vi "Differenzzeit ermitteln.vi"(9 "Zeitstempel 2":timestamp, 11 "Zeitstempel 1":timestamp) -> (1 "Differenzzeit in ms":sgl, 2 "Differenzzeit in sec":sgl)   [LabVIEW 2020, in "LogKonfig.lvlib"]
uses:
  LogKonfig.lvlib
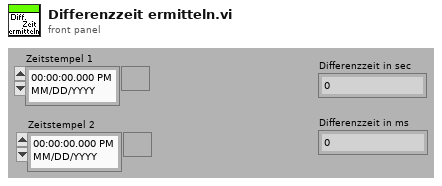
[diagram p1: front panel]
types:
  T1 = typedef "LVDateTimeRec.ctl" = cluster{"Sekundenbruchteil":dbl, "Sekunde":i32, "Minute":i32, "Stunde":i32, "Tag des Monats":i32, "Monat":i32, "Jahr":i32, "Wochentag":i32, "Tag des Jahres":i32, "DST":i32}
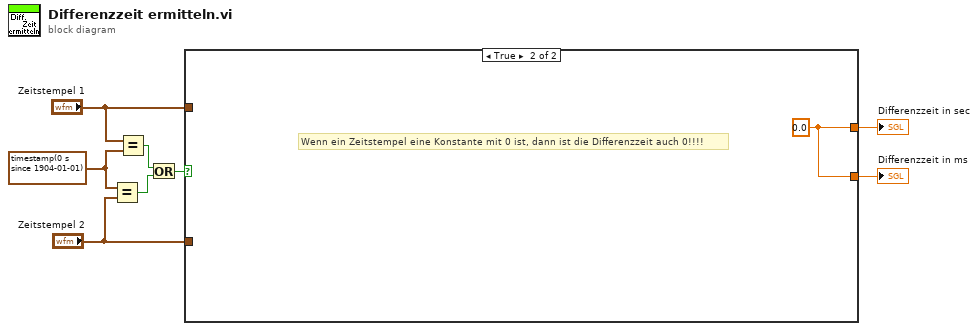
[diagram p0: block diagram]
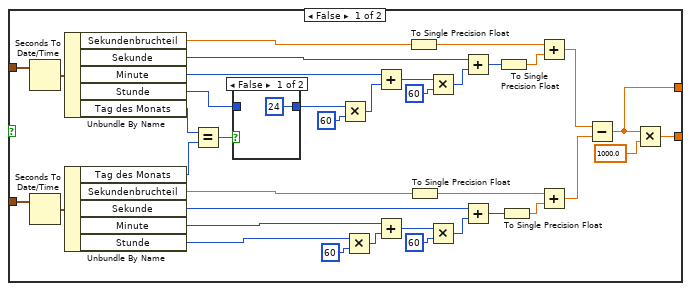
[diagram p2: hidden frame]
diagram:
  w5 = timestamp(0 s since 1904-01-01) ("Zeitstempel 2")
  n1 = Equal?(x=w5, y="Zeitstempel 2") -> (x = y?=w2:bool)
  n2 = Equal?(x="Zeitstempel 1", y=w5) -> (x = y?=w3:bool)
  n3 = Or(x=w3, y=w2) -> (x .or. y?=w1:bool)
  n4 = case shown="True" w1 {
    tunnel: [w23 w48] -> w8
    tunnel: [w21 w48] -> w7
    tunnel: "Zeitstempel 1" -> [w10 _]
    tunnel: "Zeitstempel 2" -> [w9 _]
    frame False {
      n5 = Seconds To Date/Time(time stamp (now)=w10) -> (date time rec=w44:T1)  [unwired: 1 in]
      n6 = Seconds To Date/Time(time stamp (now)=w9) -> (date time rec=w26:T1)  [unwired: 1 in]
      n7 = Unbundle By Name(w44) -> ("Sekundenbruchteil"=w12:dbl, "Sekunde"=w39:i32, "Minute"=w42:i32, "Stunde"=w20:i32, "Tag des Monats"=w16:i32)
      n8 = Unbundle By Name(w26) -> ("Tag des Monats"=w15:i32, "Sekundenbruchteil"=w14:dbl, "Sekunde"=w32:i32, "Minute"=w29:i32, "Stunde"=w18:i32)
      n9 = Equal?(x=w16, y=w15) -> (x = y?=w17:bool)
      n10 = case shown="False" w17 {
        tunnel: w20 -> [_ w47]
        tunnel: [24 ("Stunde") w47] -> w19
        frame False {
        }
        frame True {
        }
      }
      n11 = Multiply(x=w19, y=60) -> (x*y=w41:i32)
      n12 = Multiply(x=w18, y=60) -> (x*y=w30:i32)
      n13 = Add(x=w42, y=w41) -> (x+y=w40:i32)
      n14 = Add(x=w29, y=w30) -> (x+y=w31:i32)
      n15 = To Single Precision Float(number=w12) -> (single precision float=w11:sgl)
      n16 = To Single Precision Float(number=w14) -> (single precision float=w13:sgl)
      n17 = Multiply(x=w40, y=60) -> (x*y=w38:i32)
      n18 = Multiply(x=w31, y=60) -> (x*y=w33:i32)
      n19 = Add(x=w39, y=w38) -> (x+y=w37:i32)
      n20 = Add(x=w32, y=w33) -> (x+y=w34:i32)
      n21 = To Single Precision Float(number=w37) -> (single precision float=w36:sgl)
      n22 = To Single Precision Float(number=w34) -> (single precision float=w35:sgl)
      n23 = Add(x=w11, y=w36) -> (x+y=w25:sgl)
      n24 = Add(x=w13, y=w35) -> (x+y=w24:sgl)
      n25 = Subtract(x=w25, y=w24) -> (x-y=w23:sgl)
      n26 = Multiply(x=w23, y=sgl 1000.0) -> (x*y=w21:sgl)
    }
    frame True {
      w48 = sgl 0.0
      # "Wenn ein Zeitstempel eine Konstante mit 0 ist, dann ist die Differenzzeit auch 0!!!!"
    }
  }
  "Differenzzeit in ms" <- w7
  "Differenzzeit in sec" <- w8
